vi "classify error.vi"(8 "error to classify":errorcluster, 11 "Profibus Module runtime in":refnum<class "Profibus Module runtime.lvclass">) -> (0 "classified error":errorcluster, 2 "error classification":T1, 3 "Profibus Module runtime out":refnum<class "Profibus Module runtime.lvclass">)   [LabVIEW 2013, in "Profibus Module runtime.lvclass"]
doc: "Allows a module to classify an error generated at any point during execution. This <b>error classification</b> can then be used by calling code to determine if execution can continue. In addition, this function can be used to allow a component to clear an error, convert an error to a warning, or attempt to recover from an error. Recovery may be attempted only if <b>attempt recovery?</b> is true."
uses:
  Profibus Module runtime.lvclass
  <vilib>/NI/Tag Bus Module Framework/runtime/error classification.ctl
  <vilib>/NI/Tag Bus Module Framework/runtime/TBM module execution interface.lvclass
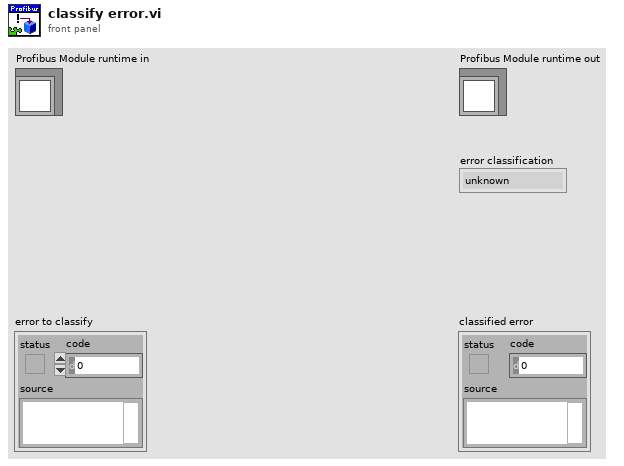
[diagram p1: front panel]
types:
  T1 = typedef "TBM module execution interface.lvclass/error classification.ctl" = enum16{"unknown", "none", "trivial", "recoverable", "critical"}
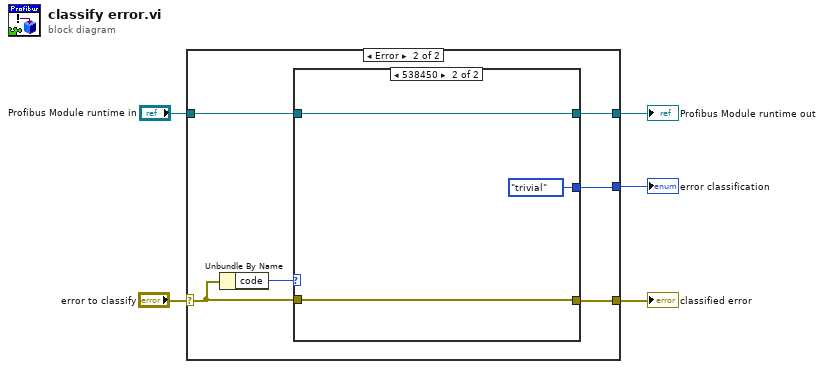
[diagram p0: block diagram]
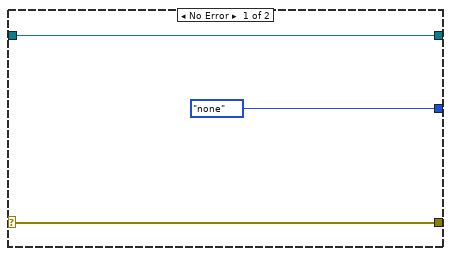
[diagram p2: hidden frame]
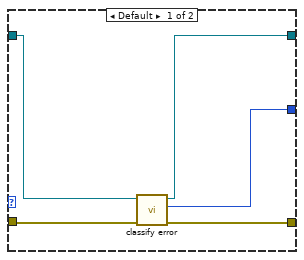
[diagram p3: hidden frame]
diagram:
  n1 = case shown="Error" "error to classify" {
    selector: "error to classify" -> [w7 w13]
    tunnel: [w8 w10] -> w4
    tunnel: "Profibus Module runtime in" -> [w8 w11]
    tunnel: [w7 w12] -> w2
    tunnel: [error_classification."none" ("error classification") w9] -> w1
    frame No Error {
    }
    frame Error {
      n2 = Unbundle By Name(w13) -> ("code"=w14:i32)
      n3 = case shown="538450" w14 {
        tunnel: w13 -> [w19 w21]
        tunnel: [w18 w21] -> w12
        tunnel: w11 -> [w17 w22]
        tunnel: [w16 w22] -> w10
        tunnel: [w15 error_classification."trivial" ("error classification")] -> w9
        frame Default {
          n4 = call-parent "classify error.vi"("error to classify"=w19, "module in"=w17) -> ("classified error"=w18:errorcluster, "error classification"=w15:T1, "module out"=w16:refnum<class "Profibus Module runtime.lvclass">)  [unwired: 7 in]
        }
        frame 538450 {
        }
      }
    }
  }
  "Profibus Module runtime out" <- w4
  "error classification" <- w1
  "classified error" <- w2
